vi "write_fifo_resonance_cross_correlate.vi"(5 "enable fly-back reversion?":bool, 6 "invert channels":bool[](array[boolean])=[FALSE, FALSE], 7 "fly-back?":bool, 8 "pixel finished?":bool, 10 "maximum bit depth":i8, 11 "integration cluster in":T1={"channel 0"=0, "channel 1"=0, "fly-back heap address"=0, "fly-forward heap address"=0, "xc buffer"=[0, 0, 0, 0, 0]}) -> (0 "FIFO overflow out":bool, 3 "integration cluster out":T1)   [LabVIEW 2010]
uses:
  integration_cluster.ctl
  <vilib>/rvi/DataTransferAndStorage/Container/XNode/niFpgaContainer.xnode
  <vilib>/rvi/DataTransferAndStorage/Container/Common/niFpgaContainerMethod.ctl
  <vilib>/rvi/DataTransferAndStorage/Container/Common/niFpgaTransferTypeControl.ctl
  <vilib>/rvi/Memory/Memory_Emulation/nirvimemoryEmulationManagerCache_GetValue.vi
  <vilib>/rvi/DataTransferAndStorage/Container/Common/niFpgaContainerGetUniqueNameForEmu.vi
  <vilib>/rvi/Memory/Memory_Emulation/nirvimemoryEmulationManagerCache_InsertValue.vi
  <vilib>/Utility/error.llb/Clear Errors.vi
  <vilib>/rvi/Memory/Memory_Emulation/nirvimemoryEmulationManagerCache_SetValue.vi
  <vilib>/rvi/interface/RandomDataEmulation/nirviRandomDataFPGAFIFO.vi
  <vilib>/rvi/interface/RandomDataEmulation/niFpgaRandomDataHandleErrors.vi
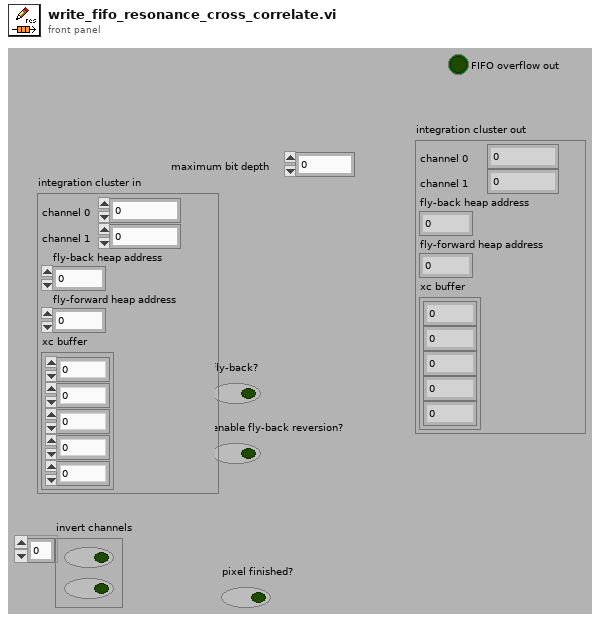
[diagram p1: front panel]
types:
  T1 = typedef "integration_cluster.ctl" = cluster{"channel 0":u32, "channel 1":u32, "fly-back heap address":u32, "fly-forward heap address":u32, "xc buffer":u32[]}
  T2 = typedef "niFpgaContainerMethod.ctl" = enum16{"<none>", "write", "read", "clear", "getNumberOfElementsToWrite", "getNumberOfElementsToRead", "enable", "disable", "flushAndDisable", "getStreamState", "readA", "readB", "dramWrite", "dramWriteWithByteEnables", "dramRequestData", "dramRetrieveData"}
  T3 = typedef "niFpgaTransferTypeControl.ctl" = enum16{"Target-Scoped", "Host to Target - DMA", "Target to Host - DMA", "Peer to Peer Reader", "Peer to Peer Writer", "Bidirectional"}
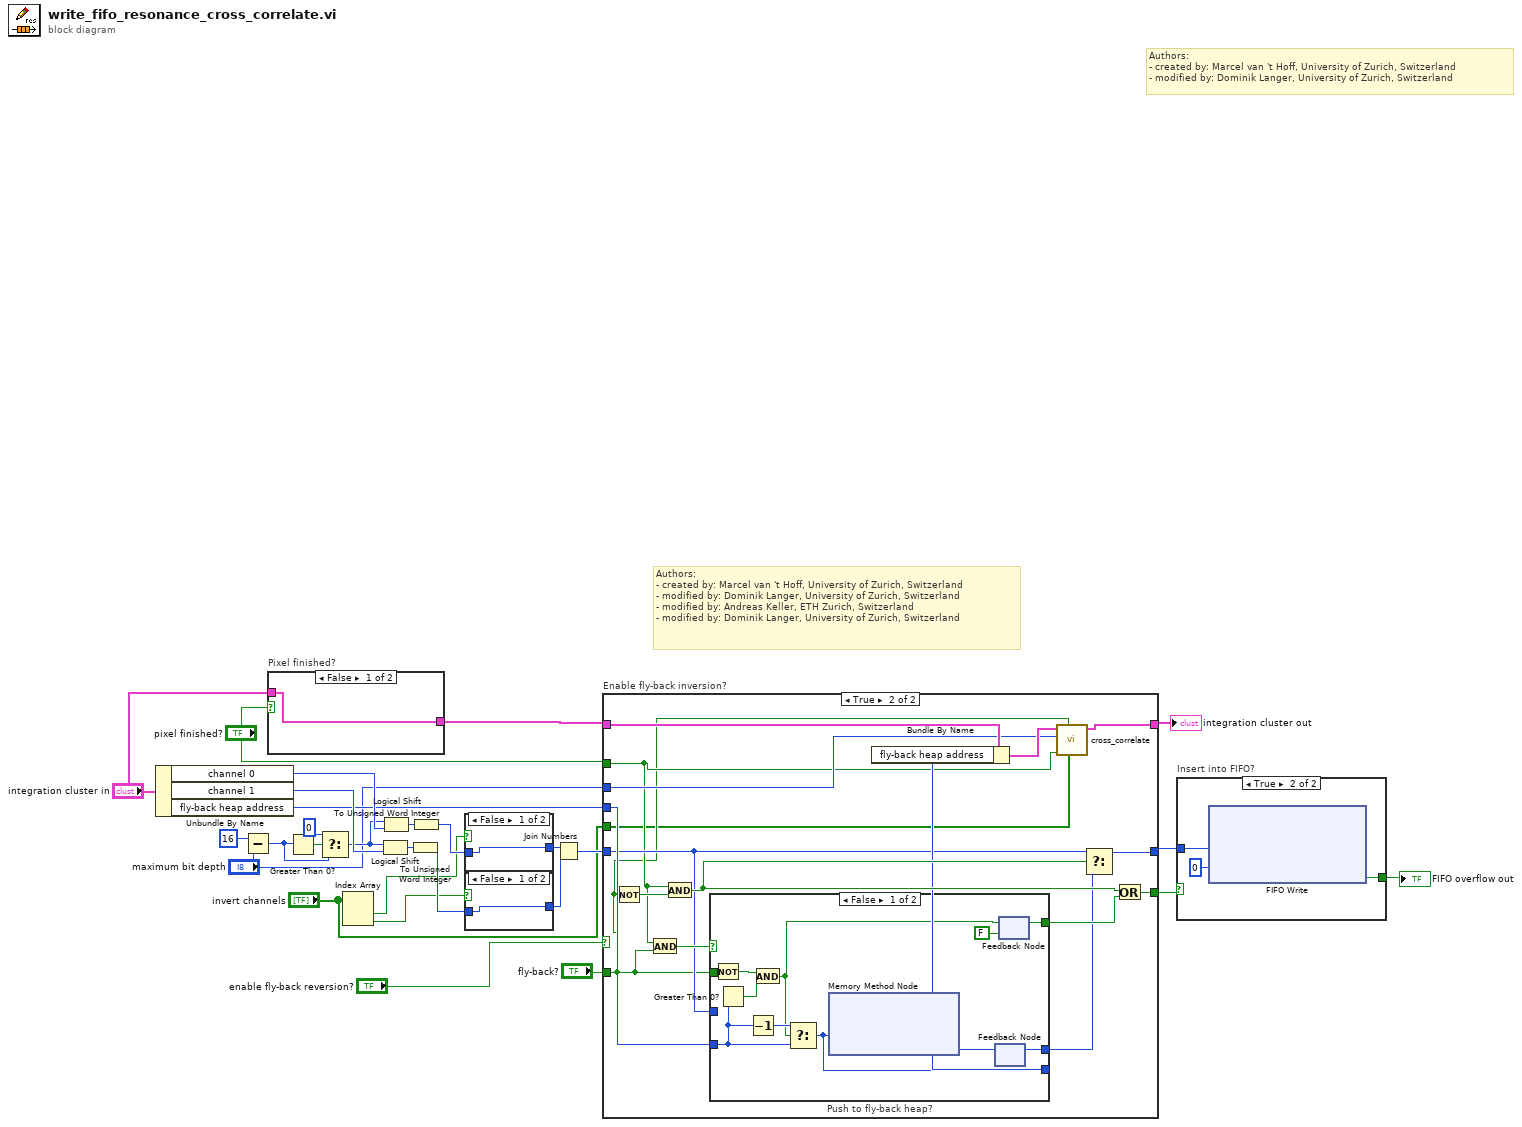
[diagram p0: block diagram]
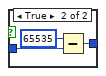
[diagram p2: hidden frame]
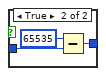
[diagram p3: hidden frame]
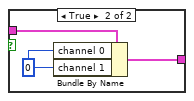
[diagram p4: hidden frame]
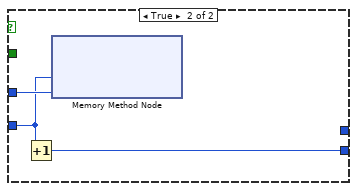
[diagram p6: hidden frame]
diagram:
  # "Authors: \n- created by: Marcel van 't Hoff, University of Zurich, Switzerland\n- modified by: Dominik Langer, University of Zurich, Switzerland\n- modified by: Andreas Keller, ETH Zurich, Switzerland\n- modified by: Dominik Langer, University of Zurich, Switzerland"
  # "Authors: \n- created by: Marcel van 't Hoff, University of Zurich, Switzerland\n- modified by: Dominik Langer, University of Zurich, Switzerland"
  n1 = Unbundle By Name("integration cluster in") -> ("channel 0"=w22:u32, "channel 1"=w23:u32, "fly-back heap address"=w14:u32)
  n2 = Subtract(x=i8 16, y="maximum bit depth") -> (x-y=w25:i8)
  n3 = case "Pixel finished?" shown="False" "pixel finished?" {
    tunnel: "integration cluster in" -> [w29 w31]
    tunnel: [w29 w30] -> w11
    frame False {
    }
    frame True {
      w32 = u32 0 ("channel 1")
      n4 = Bundle By Name(cluster=w31, "channel 0"=w32, "channel 1"=w32) -> (w30:T1)
    }
  }
  n5 = Greater Than 0?(x=w25) -> (x > 0?=w24:bool)
  n6 = Select(t=i8 0 ("f"), s=w24, f=w25) -> (s? t:f=w21:i8)
  n7 = Index Array(array="invert channels") -> (element #1=w4:bool, element #2=w3:bool)  [unwired: 2 in]
  n8 = Logical Shift(y=w21, x=w23) -> (x << y=w20:u32)
  n9 = Logical Shift(y=w21, x=w22) -> (x << y=w19:u32)
  n10 = To Unsigned Word Integer(number=w20) -> (unsigned 16bit integer=w6:u16)
  n11 = To Unsigned Word Integer(number=w19) -> (unsigned 16bit integer=w8:u16)
  n12 = case shown="False" w4 {
    tunnel: [w33 w35] -> w7
    tunnel: w8 -> [w33 w34]
    frame False {
    }
    frame True {
      n13 = Subtract(x=u16 65535, y=w34) -> (x-y=w35:u16)
    }
  }
  n14 = case shown="False" w3 {
    tunnel: [w37 w39] -> w5
    tunnel: w6 -> [w37 w38]
    frame False {
    }
    frame True {
      n15 = Subtract(x=u16 65535, y=w38) -> (x-y=w39:u16)
    }
  }
  n16 = Join Numbers(hi=w7, lo=w5) -> ((hi.lo)=w18:u32)
  n17 = case "Enable fly-back inversion?" shown="True" "enable fly-back reversion?" {
    tunnel: w14 -> [_ w60]
    tunnel: w18 -> [w43 w52]
    tunnel: [w43 w58] -> w17
    tunnel: "pixel finished?" -> [w42 w47]
    tunnel: [w42 w51] -> w13
    tunnel: "fly-back?" -> [_ w46]
    tunnel: w11 -> [w41 w54]
    tunnel: [w41 w44] -> w9
    tunnel: "maximum bit depth" -> [_ w48]
    tunnel: "invert channels" -> [_ w45]
    frame False {
    }
    frame True {
      n18 = Not(x=w46) -> (.not. x?=w59:bool)
      n19 = And(x=w47, y=w46) -> (x .and. y?=w57:bool)
      n20 = And(x=w47, y=w59) -> (x .and. y?=w56:bool)
      n21 = case "Push to fly-back heap?" shown="False" w57 {
        tunnel: w52 -> [_ w200]
        tunnel: [w63 w199] -> w53
        tunnel: w60 -> [w65 w198]
        tunnel: w46 -> [w70 _]
        tunnel: [w67 _] -> w50
        tunnel: [w69 _] -> w55
        frame False {
          n22 = Not(x=w70) -> (.not. x?=w62:bool)
          n23 = Greater Than 0?(x=w65) -> (x > 0?=w71:bool)
          n24 = Decrement(x=w65) -> (x-1=w64:u32)
          n25 = And(x=w62, y=w71) -> (x .and. y?=w61:bool)
          n26 = Select(t=w64, s=w61, f=w65) -> (s? t:f=w63:u32)
          n27 = xnode ("Memory Method Node")("Address"=w63) -> ("Data"=w66:u32)  [unwired: 1 in, 1 out]
          n28 = feedback #1() -> (w67:u32)  [unwired: 1 in]
          n29 = feedback-in #1(w66) -> ()
          n30 = feedback #2(FALSE) -> (w69:bool)
          n31 = feedback-in #2(w61) -> ()
        }
        frame True {
          n32 = Increment(x=w198) -> (x+1=w199:u32)
          n33 = xnode ("Memory Method Node")("Address"=w198, "Data"=w200) -> ()  [unwired: 1 in, 1 out]
        }
      }
      n34 = Bundle By Name(cluster=w54, "fly-back heap address"=w53) -> (w49:T1)
      n35 = call "cross_correlate.vi"("invert channels"=w45, "fly-back?"=w46, "pixel finished?"=w47, "maximum bit depth"=w48, "integration cluster in"=w49) -> ("integration cluster out"=w44:T1)  [unwired: 6 in]
      n36 = Select(t=w52, s=w56, f=w50) -> (s? t:f=w58:u32)
      n37 = Or(x=w56, y=w55) -> (x .or. y?=w51:bool)
    }
  }
  "integration cluster out" <- w9
  n38 = case "Insert into FIFO?" shown="True" w13 {
    tunnel: [_ w328] -> w28
    tunnel: w17 -> [_ w326]
    frame False {
    }
    frame True {
      n39 = xnode ("FIFO Write")("Element"=w326, "Timeout"=0) -> ("Timed Out?"=w328:bool)  [unwired: 1 in, 1 out]
    }
  }
  "FIFO overflow out" <- w28
